vi "Unit Test.vi"() -> ()   [LabVIEW 2017]
uses:
  Oven/Custom Controls/Message Type.ctl
  Oven/Oven.lvclass
  Oven/Oven.lvlib
panel:
  in  "Oven State:":bool
  in  "Temperature Setpoint":dbl
  in  "stop":bool
  out "Read Data":u8[](array[numeric]) format="%.0x"
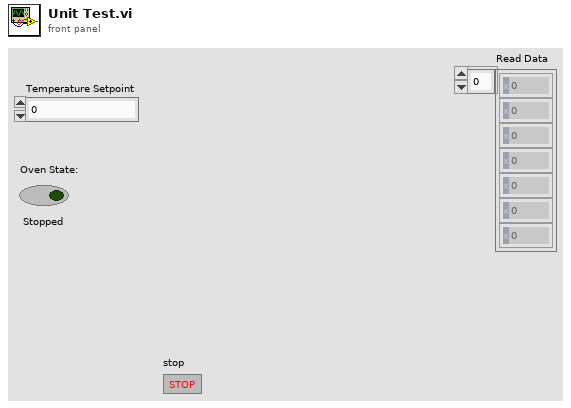
[diagram p1: front panel]
types:
  T1 = typedef "Oven.lvlib/Message Type.ctl" = enum16{"Start", "Stop", "Set Temperature", "Get Temperature"}
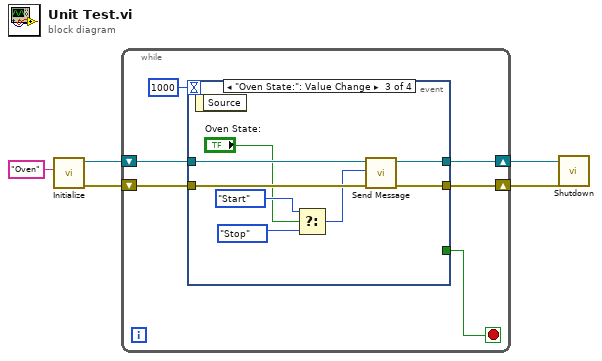
[diagram p0: block diagram]
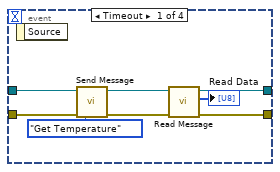
[diagram p2: hidden frame]
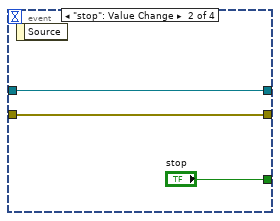
[diagram p3: hidden frame]
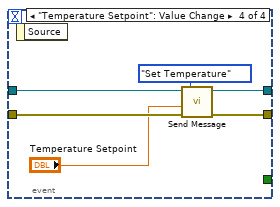
[diagram p4: hidden frame]
diagram:
  n1 = call "Initialize.vi"("Device"="Oven") -> ("error out"=w3:errorcluster, "Oven out"=w4:refnum<class "Oven.lvclass">)  [unwired: 9 in]
  n2 = while {
    shift-right: [w8] -> w1
    shift-left: w4 -> [w10]
    shift-right: [w7] -> w2
    shift-left: w3 -> [w9]
    stop <- w6 stop-if-true
    n3 = event shown="[2] \"Oven State:\": Value Change" {
      selector: _ -> [_ _ _ _]
      dyn-events: _ -> [_ _ _ _]
      timeout: 1000 -> [_ _ _ _]
      tunnel: w10 -> [w19 w22 w29 w36]
      tunnel: w9 -> [w18 w21 w30 w33]
      tunnel: [w15 w22 w28 w35] -> w8
      tunnel: [w14 w21 w27 w34] -> w7
      tunnel: [_ "stop" _ _] -> w6
      event Timeout {
        n4 = event-data() -> ()  [unwired: 1 in, 1 out]
        n5 = call-dynamic "Send Message.vi"("error in (no error)"=w18, "Message to Send"=Message_Type."Get Temperature", "Oven in"=w19) -> ("error out"=w17:errorcluster, "Oven out"=w16:refnum<class "Oven.lvclass">)  [unwired: 7 in]
        n6 = call-dynamic "Read Message.vi"("error in (no error)"=w17, "Oven in"=w16) -> ("error out"=w14:errorcluster, "Array"=→"Read Data":u8[], "Oven out"=w15:refnum<class "Oven.lvclass">)  [unwired: 7 in]
      }
      event "stop": Value Change {
        n7 = event-data() -> ()  [unwired: 1 in, 1 out]
      }
      event "Oven State:": Value Change {
        n8 = event-data() -> ()  [unwired: 1 in, 1 out]
        n9 = Select(t=Message_Type."Start" ("Message to Send"), s="Oven State:", f=Message_Type."Stop" ("Message to Send")) -> (s? t:f=w23:T1)
        n10 = call-dynamic "Send Message.vi"("error in (no error)"=w30, "Message to Send"=w23, "Oven in"=w29) -> ("error out"=w27:errorcluster, "Oven out"=w28:refnum<class "Oven.lvclass">)  [unwired: 7 in]
      }
      event "Temperature Setpoint": Value Change {
        n11 = event-data() -> ()  [unwired: 1 in, 1 out]
        n12 = call-dynamic "Send Message.vi"("error in (no error)"=w33, "Value"="Temperature Setpoint", "Message to Send"=Message_Type."Set Temperature", "Oven in"=w36) -> ("error out"=w34:errorcluster, "Oven out"=w35:refnum<class "Oven.lvclass">)  [unwired: 6 in]
      }
    }
  }
  n13 = call "Shutdown.vi"("error in"=w2, "Oven in"=w1) -> ()  [unwired: 8 in, 2 out]
